vi "close_DAQmx_ports.vi"(8 "error in (no error)":errorcluster, 10 "task/channels in 2":refnum<k21>, 11 "task/channels in 1":refnum<k21>) -> (0 "error out":errorcluster)   [LabVIEW 2015]
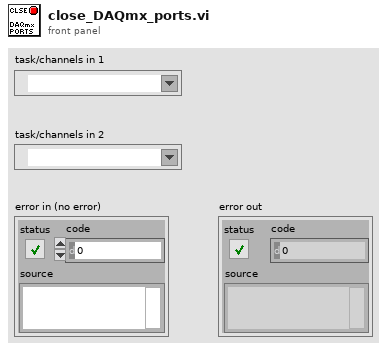
[diagram p1: front panel]
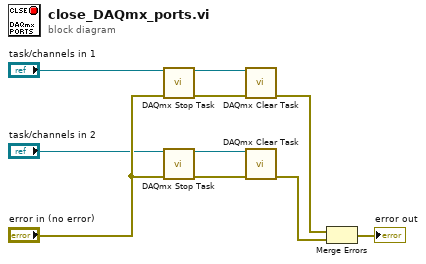
[diagram p0: block diagram]
diagram:
  n1 = call <vilib>:"DAQmx Stop Task.vi"("task/channels in"="task/channels in 1", "error in"="error in (no error)") -> ("task out"=w9:refnum<k21>, "error out"=w10:errorcluster)  [unwired: 12 in]
  n2 = call <vilib>:"DAQmx Stop Task.vi"("task/channels in"="task/channels in 2", "error in"="error in (no error)") -> ("task out"=w8:refnum<k21>, "error out"=w7:errorcluster)  [unwired: 12 in]
  n3 = call <vilib>:"DAQmx Clear Task.vi"("task in"=w9, "error in"=w10) -> ("error out"=w5:errorcluster)  [unwired: 13 in]
  n4 = call <vilib>:"DAQmx Clear Task.vi"("task in"=w8, "error in"=w7) -> ("error out"=w4:errorcluster)  [unwired: 13 in]
  n5 = Merge Errors(w5, w4) -> (→"error out":errorcluster)
